vi "Last Ack Creator Queue.vi"(10 "Queue":refnum<class "Queue.lvclass">, 11 "jettl Msg Last Ack Creator Queue in":refnum<class "jettl Msg Last Ack Creator Queue.lvclass">) -> (3 "jettl Msg Last Ack Creator Queue out":refnum<class "jettl Msg Last Ack Creator Queue.lvclass">)   [LabVIEW 2021, in "jettl.lvlib" / "Last Ack Creator Queue Msg Strategy.lvlib" / "jettl Msg Last Ack Creator Queue.lvclass"]
uses:
  jettl Msg Last Ack Creator Queue.lvclass
  Queue/Queue.lvclass
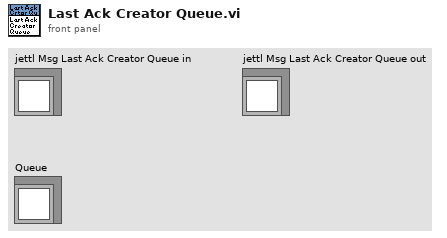
[diagram p1: front panel]
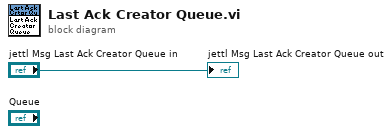
[diagram p0: block diagram]
diagram:
  "jettl Msg Last Ack Creator Queue out" <- "jettl Msg Last Ack Creator Queue in"
